vi "Create New Project.vi"(8 "error in (no error)":errorcluster, 9 "File Path to Append":path, 10 "Build Specs Folder Path":path=path "C:/sw-deps-monitor/Source/BuildSpecs", 11 "Source Folder Path":path=path "C:/sw-deps-monitor/Source") -> (0 "error out":errorcluster, 1 "Project Mismatch Path":path, 2 "ExpectedDeps Files Created":path, 3 "Project Created":path, 4 "Project Path Mismatch?":bool, 5 "Owned Class[]":path[](array[path]))   [LabVIEW 2019, in "DepsWatch.lvlib"]
uses:
  DepsWatch.lvlib
  <userlib>/_OpenG.lib/file/file.llb/Append Path to Root if Relative - Scalar__ogtk.vi
  <userlib>/_OpenG.lib/file/file.llb/Compare Two Paths - Scalar__ogtk.vi
  <userlib>/_OpenG.lib/file/file.llb/File Exists - Scalar__ogtk.vi
  <vilib>/Utility/config.llb/NI_LVConfig.lvlib
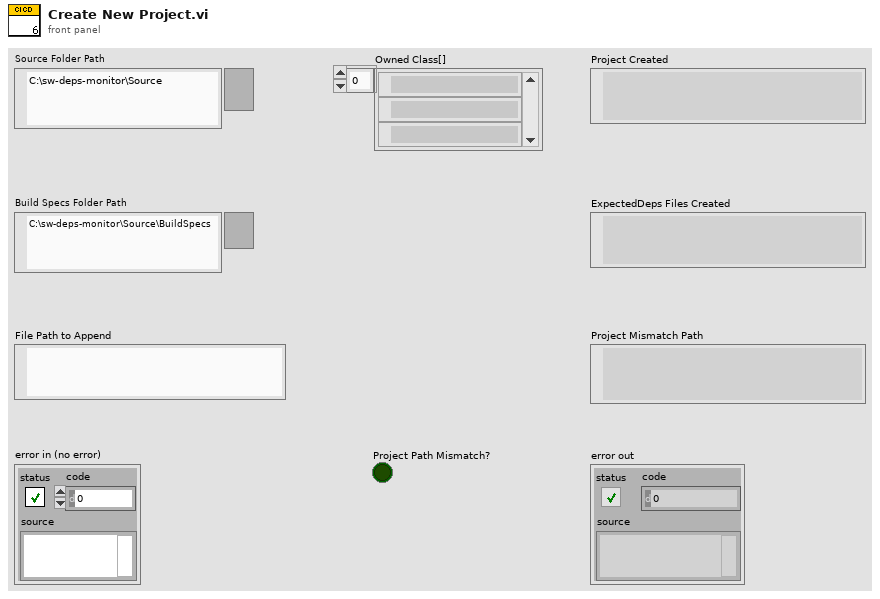
[diagram p1: front panel]
types:
  T1 = typedef "NI_LVConfig.lvlib/Config Data RefNum.ctl" = refnum<k1>
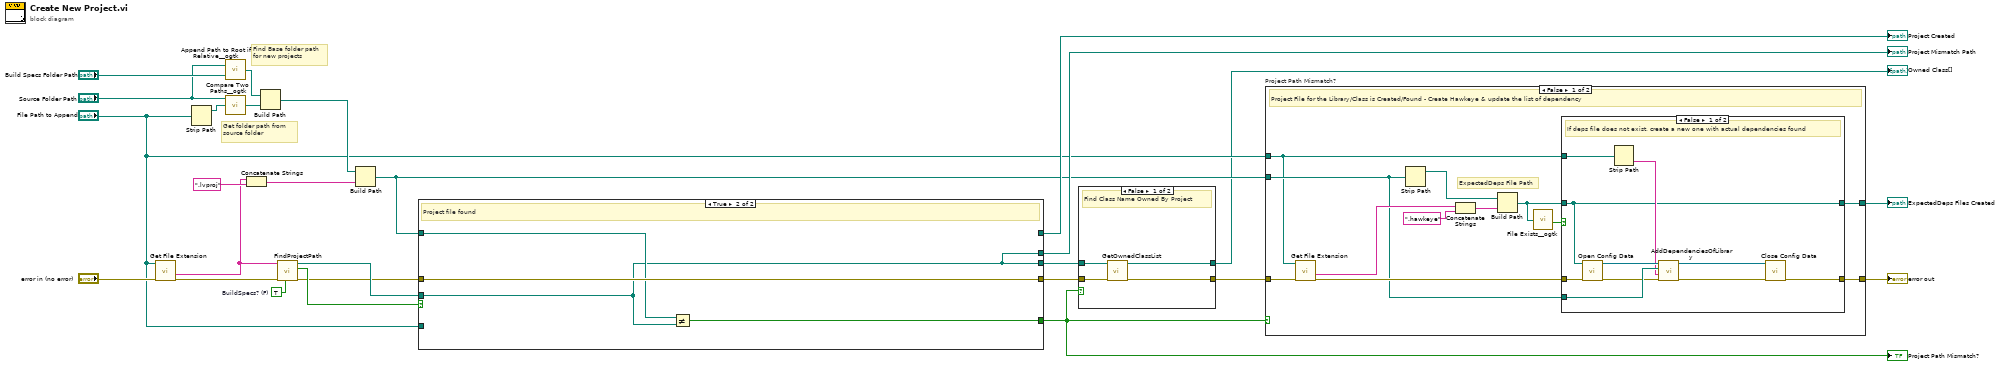
[diagram p0: block diagram]
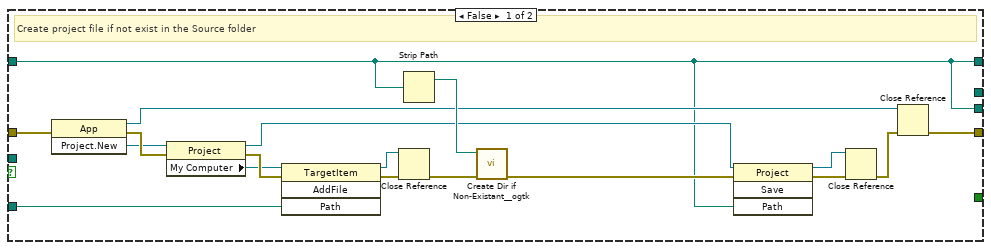
[diagram p5: hidden frame]
diagram:
  w19 = TRUE  # BuildSpecs? (F)
  # "Find Base folder path for new projects"
  # "Get folder path from source folder"
  n1 = call <vilib>:"Get File Extension.vi"("error in (no error)"="error in (no error)", "file"="File Path to Append") -> ("error out"=w20:errorcluster, "filename without extension"=w21:string)  [unwired: 5 in, 3 out]
  n2 = Strip Path(path="File Path to Append") -> (stripped path=w18:path)  [unwired: 1 out]
  n3 = call-poly <userlib>:"Append Path to Root if Relative__ogtk.vi"("Absolute or Relative Path"="Build Specs Folder Path", "Root Path"="Source Folder Path") -> ("Absolute or Appended Path"=w17:path)
  n4 = call-poly <userlib>:"Compare Two Paths__ogtk.vi"("path2"=w18, "path1"="Source Folder Path") -> ("relative path from 1 to 2"=w16:path)  [unwired: 1 in, 2 out]
  n5 = Concatenate Strings(w21, ".lvproj" ("string")) -> (w22:string)
  n6 = Build Path(base path=w17, name or relative path=w16) -> (appended path=w12:path)
  n7 = call "FindProjectPath.vi"("BuildSpecs? (F)"=w19, "error in (no error)"=w20, "Library/Class Name"=w21) -> ("error out"=w13:errorcluster, "Found?"=w15:bool, "Project Path"=w14:path)  [unwired: 6 in]
  n8 = Build Path(base path=w12, name or relative path=w22) -> (appended path=w8:path)
  n9 = case shown="True" w15 {
    tunnel: [w43 w48] -> w5
    tunnel: "File Path to Append" -> [w44 _]
    tunnel: w13 -> [w42 w48]
    tunnel: w8 -> [w27 w46]
    tunnel: w14 -> [_ w45]
    tunnel: [_ w47] -> w3
    tunnel: [_ w45] -> w11
    tunnel: [w27 _] -> w10
    tunnel: [w27 w45] -> w2
    frame False {
      # "Create project file if not exist in the Source folder"
      n10 = invoke class="App" method="Project.New"(error in=w42) -> (reference out=w29:refnum<vi>, error out=w30:errorcluster, "Project:New"=w28:refnum<vi>)  [unwired: 2 in]
      n11 = property class="Project"(reference=w28, error in=w30) -> (reference out=w36:refnum<vi>, error out=w32:errorcluster, "My Computer"=w31:refnum<vi>)
      n12 = invoke class="TargetItem" method="AddFile"(reference=w31, error in=w32, "Path"=w44) -> (reference out=w33:refnum<vi>, error out=w34:errorcluster)  [unwired: 1 in, 2 out]
      n13 = Close Reference(reference=w33, error in (no error)=w34) -> (error out=w39:errorcluster)
      n14 = Strip Path(path=w27) -> (stripped path=w41:path)  [unwired: 1 out]
      n15 = call <userlib>:"Create Dir if Non-Existant__ogtk.vi"("error in (no error)"=w39, "Directory Path"=w41) -> ("error out"=w40:errorcluster)  [unwired: 7 in, 2 out]
      n16 = invoke class="Project" method="Save"(reference=w36, error in=w40, "Path"=w27) -> (reference out=w37:refnum<vi>, error out=w38:errorcluster)  [unwired: 1 in, 2 out]
      n17 = Close Reference(reference=w37, error in (no error)=w38) -> (error out=w35:errorcluster)
      n18 = Close Reference(reference=w29, error in (no error)=w35) -> (error out=w43:errorcluster)
    }
    frame True {
      # "Project file found"
      n19 = Not Equal?(x=w46, y=w45) -> (x != y?=w47:bool)
    }
  }
  "Project Path Mismatch?" <- w3
  "Project Mismatch Path" <- w11
  "Project Created" <- w10
  n20 = case shown="False" w3 {
    tunnel: w5 -> [w52 w53]
    tunnel: [w51 w53] -> w4
    tunnel: w2 -> [w50 _]
    tunnel: [w49 _] -> w1
    frame False {
      # "Find Class Name Owned By Project"
      n21 = call "GetOwnedClassList.vi"("error in (no error)"=w52, "Project Path"=w50) -> ("error out"=w51:errorcluster, "Owned Class[]"=w49:path[])  [unwired: 8 in]
    }
    frame True {
    }
  }
  "Owned Class[]" <- w1
  n22 = case "Project Path Mismatch?" shown="False" w3 {
    tunnel: w4 -> [w65 w77]
    tunnel: [w64 w77] -> w9
    tunnel: w8 -> [w56 _]
    tunnel: "File Path to Append" -> [w55 _]
    tunnel: [w54 _] -> w6
    frame False {
      # "ExpectedDeps File Path"
      # "Project File for the Library/Class is Created/Found - Create Hawkeye & update the list of dependency"
      n23 = call <vilib>:"Get File Extension.vi"("error in (no error)"=w65, "file"=w55) -> ("error out"=w63:errorcluster, "filename without extension"=w61:string)  [unwired: 5 in, 3 out]
      n24 = Strip Path(path=w56) -> (stripped path=w60:path)  [unwired: 1 out]
      n25 = Concatenate Strings(w61, ".hawkeye" ("string")) -> (w59:string)
      n26 = Build Path(base path=w60, name or relative path=w59) -> (appended path=w62:path)
      n27 = call-poly <userlib>:"File Exists__ogtk.vi"("file path"=w62) -> ("exists"=w57:bool)  [unwired: 6 in, 1 out]
      n28 = case shown="False" w57 {
        tunnel: w56 -> [w75 _]
        tunnel: w63 -> [w74 w76]
        tunnel: w62 -> [w66 _]
        tunnel: [w69 w76] -> w64
        tunnel: w55 -> [w67 _]
        tunnel: [w66 _] -> w54
        frame False {
          # "If deps file does not exist, create a new one with actual dependencies found"
          n29 = call <vilib>:"Open Config Data.vi"("error in (no error)"=w74, "configuration file path"=w66) -> ("error out"=w73:errorcluster, "refnum"=w72:T1)  [unwired: 7 in, 1 out]
          n30 = Strip Path(path=w67) -> (name=w68:string)  [unwired: 1 out]
          n31 = call "AddDependenciesOfLibrary.vi"("error in (no error)"=w73, "LibraryName"=w68, "Project Path"=w75, "Config Refnum in"=w72) -> ("error out"=w71:errorcluster, "Config Refnum out"=w70:T1)  [unwired: 4 in, 2 out]
          n32 = call <vilib>:"Close Config Data.vi"("error in (no error)"=w71, "refnum"=w70) -> ("error out"=w69:errorcluster)  [unwired: 8 in, 1 out]
        }
        frame True {
        }
      }
    }
    frame True {
    }
  }
  "error out" <- w9
  "ExpectedDeps Files Created" <- w6
